vi "record_to_tsv.vi"(7 "folder_name":string="anneal_tc", 8 "T1":dbl, 9 "T0":dbl, 10 "time":timestamp, 11 "file_name":string="record") -> ()   [LabVIEW 2019]
uses:
  <vilib>/Utility/file.llb/Write Delimited Spreadsheet (string).vi
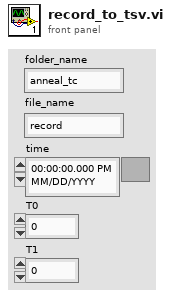
[diagram p1: front panel]
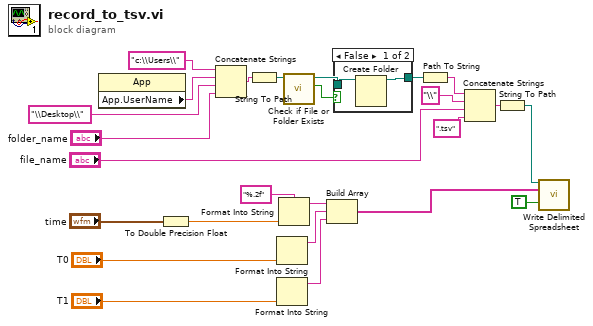
[diagram p0: block diagram]
diagram:
  n1 = property class="App"() -> ("App.UserName"=w20:string)  [unwired: 2 in, 2 out]
  n2 = To Double Precision Float(number="time") -> (double precision float=w2:dbl)
  n3 = Concatenate Strings("c:\\Users\\", w20, "\\Desktop\\", "folder_name") -> (w18:string)
  n4 = String To Path(string=w18) -> (path=w13:path)
  n5 = Format Into String("T0") -> (resulting string=w24:string)  [unwired: 3 in, 1 out]
  n6 = Format Into String("T1") -> (resulting string=w5:string)  [unwired: 3 in, 1 out]
  n7 = Format Into String(format string="%.2f", w2) -> (resulting string=w25:string)  [unwired: 2 in, 1 out]
  n8 = call <vilib>:"Check if File or Folder Exists.vi"("path"=w13) -> ("file or folder exists?"=w12:bool, "dup path"=w10:path)  [unwired: 8 in, 1 out]
  n9 = Build Array(w25, w24, w5) -> (w23:string[])
  n10 = case shown="False" w12 {
    tunnel: w10 -> [w27 w28]
    tunnel: [w26 w28] -> w11
    frame False {
      n11 = Create Folder(path (use dialog)=w27) -> (created path=w26:path)  [unwired: 2 in, 2 out]
    }
    frame True {
    }
  }
  n12 = Path To String(path=w11) -> (string=w9:string)
  n13 = Concatenate Strings(w9, "\\", "file_name", ".tsv" ("string")) -> (w14:string)
  n14 = String To Path(string=w14) -> (path=w8:path)
  n15 = call-poly <vilib>:"Write Delimited Spreadsheet.vi"("file path (dialog if empty)"=w8, "1D data"=w23, "append to file? (new file:F)"=TRUE) -> ()  [unwired: 11 in, 2 out]
